vi "Measure.vi"(8 "error in (no error)":errorcluster, 9 "measurement configuration":variant, 10 "measure call context in":refnum<class "Measure Call Context.lvclass">, 11 "measurement plugin in":refnum<class "FPT Pulse Measurement.lvclass">) -> (0 "error out":errorcluster, 1 "measurement results":variant, 2 "measure call context out":refnum<class "Measure Call Context.lvclass">, 3 "measurement plugin out":refnum<class "FPT Pulse Measurement.lvclass">)   [LabVIEW 2023, in "FPT Pulse Measurement.lvclass"]
uses:
  FPT Pulse Measurement.lvclass
  <vilib>/Plug-In SDKs/Measurements/Measure Call Context/Measure Call Context.lvclass
  Measurement Configuration.ctl
  FPT Pulse Measurement.lvclass/FPT Pulse Measurement.ctl
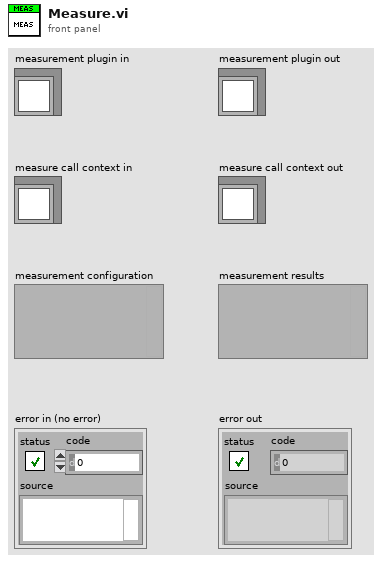
[diagram p1: front panel]
types:
  T1 = typedef "FPT Pulse Measurement.lvclass/Measurement Configuration.ctl" = cluster{"Automation Test":bool, "Power sequencing file path":string, "RFSG name":string, "RFSG port":string, "RFSG attenuation mode":enum32{"<None>", "Constant Attenuation", "s2p File"}, "RFSG external attenuation (dB)":dbl, "RFSG s-parameters orientation":enum32{"Port1 Towards DUT", "Port2 Towards DUT"}, "RFSG s2p file path":string, "RFmx name":string, "RFmx port":string, "RFmx attenuation mode":enum32{"<None>", "Constant Attenuation", "s2p File"}, "RFmx external attenuation (dB)":dbl, "RFmx s-parameters orientation":enum32{"Port1 Towards DUT", "Port2 Towards DUT"}, "RFmx s2p file path":string, "RFmx Center Frequency (Hz)":dbl, "RFmx Measurement Bandwidth (Hz)":dbl, "RFmx Reference Level (dBm)":dbl, "RFSG Generation IQ Rate (S/s)":dbl, "Pulse Acquisition Length (s)":dbl, "Pulse Power Level (dBm)":dbl, "Pulse Repetition Interval [PRI] (s)":dbl, "Pulse Width (s)":dbl, "Number of Pulses per Burst":u32, "Measurement Offset":i32, "Window Start (%)":dbl, "Window Stop (%)":dbl, "Window Step Size (%)":dbl, "High Reference Level (%)":dbl, "Width Reference Level (%)":dbl, "Low Reference Level (%)":dbl, "Selected Pulse Trace":i32, "Power sequencing file validity check":bool}
  T2 = typedef "FPT Pulse Measurement.lvclass/Measurement Results.ctl" = cluster{"Status":string, "TS Intrapulse Stability":dbl[][], "TS P2P Stability":dbl[][], "TS Acquired Amplitude":dbl[][], "Per Pulse Result":dbl[][], "Per Pulse Result (Name)":string[], "Duty Cycle (%)":dbl, "Rising Time (us)":dbl, "Fall Time (us)":dbl, "Droop (%)":dbl, "Ripple (%)":dbl, "Overshoot (%)":dbl, "Amplitude Stability (dB)":dbl, "Phase Stability (dB)":dbl}
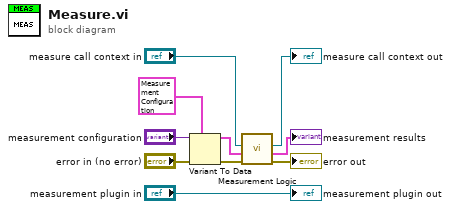
[diagram p0: block diagram]
diagram:
  n1 = Variant To Data(error in="error in (no error)", type=T1 {"Automation Test"=FALSE, "Power sequencing file path"="Lorem ipsum dolor sit", "RFSG name"="5842_0", "RFSG port"="", "RFSG attenuation mode"=enum."s2p File", "RFSG external attenuation (dB)"=64.0, "RFSG s-parameters orientation"=enum."Port1 Towards DUT", "RFSG s2p file path"="", "RFmx name"="Lorem ipsum dolor sit", "RFmx port"="", "RFmx attenuation mode"=enum."Constant Attenuation", "RFmx external attenuation (dB)"=-64.0, "RFmx s-parameters orientation"=enum."Port2 Towards DUT", "RFmx s2p file path"="", "RFmx Center Frequency (Hz)"=10000000000.0, "RFmx Measurement Bandwidth (Hz)"=80000000.0, "RFmx Reference Level (dBm)"=10.0, "RFSG Generation IQ Rate (S/s)"=10000000000.0, "Pulse Acquisition Length (s)"=80000000.0, "Pulse Power Level (dBm)"=10.0, "Pulse Repetition Interval [PRI] (s)"=1250000000.0, "Pulse Width (s)"=0.001, "Number of Pulses per Burst"=0, "Measurement Offset"=0, "Window Start (%)"=2e-05, "Window Stop (%)"=20.0, "Window Step Size (%)"=0.0, "High Reference Level (%)"=10.0, "Width Reference Level (%)"=90.0, "Low Reference Level (%)"=10.0, "Selected Pulse Trace"=0, "Power sequencing file validity check"=FALSE} ("measurement configuration"), Variant="measurement configuration") -> (data=w1:T1, error out=w7:errorcluster)
  n2 = call "Measurement Logic.vi"("error in"=w7, "measurement configuration"=w1, "measure call context in"="measure call context in") -> ("error out"=→"error out":errorcluster, "measurement results"=→"measurement results":T2, "measure call context out"=→"measure call context out":refnum<class "Measure Call Context.lvclass">)  [unwired: 6 in]
  "measurement plugin out" <- "measurement plugin in"
